vi "Write IO_EN VIS.vi"(8 "error in":errorcluster, 10 "Visible":bool, 11 "DIG_IO in":refnum<class "DIG_IO.lvclass">) -> (0 "error out":errorcluster, 3 "DIG_IO out":refnum<class "DIG_IO.lvclass">)   [LabVIEW 2019, in "DIG_IO.lvlib" / "DIG_IO.lvclass"]
uses:
  Library/DIG_IO.lvclass
  Library/DIG_IO.lvclass/DIG_IO.ctl
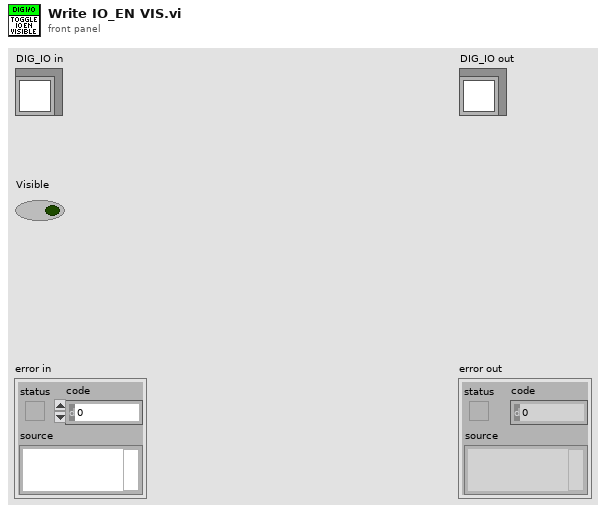
[diagram p1: front panel]
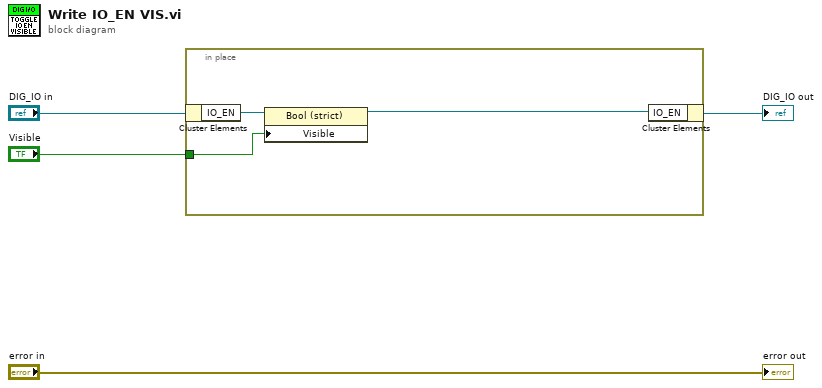
[diagram p0: block diagram]
diagram:
  n1 = in-place {
    in-place-border: "Visible" -> [w5]
    n2 = in-place-cluster #1("DIG_IO in") -> ("IO_EN"=w7:refnum<vi>)
    n3 = property class="Bool (strict)"(reference=w7, "Visible"=w5) -> (reference out=w6:refnum<vi>)  [unwired: 1 in, 1 out]
    n4 = in-place-cluster #1("IO_EN"=w6) -> (→"DIG_IO out":refnum<class "DIG_IO.lvclass">)
  }
  "error out" <- "error in"
